vi "Write Custom Serialization Binder Then Read - Returns Same Object.vi"() -> ()   [LabVIEW 2017, in "Generic Object Serializer Tests.lvlib" / "Serialization Binder.lvlib"]
uses:
  Serialization Binder.lvlib
  Generic Object Serializer/Generic Object Serializer.lvclass
  Error Serialization Binder/Error Serialization Binder.lvclass
  C:/Users/de200256/Code/logmanoriginal/jsontext-object-serialization/Serialization Binder/Serialization Binder.lvclass
  Generic Object Serializer/Generic Object Serializer.lvclass/Generic Object Serializer.ctl
  Generic Object Serializer/Write Serialization Binder.vi
  Generic Object Serializer/Read Serialization Binder.vi
  Default Serialization Binder/Default Serialization Binder.lvclass
  Serialization Binder/Serialization Binder.lvclass
  <vilib>/addons/_JKI Toolkits/Caraya/classes/Assert/Assert.lvclass
  <vilib>/addons/_JKI Toolkits/Caraya/classes/Test/Test.lvclass
panel:
  out "error out":errorcluster
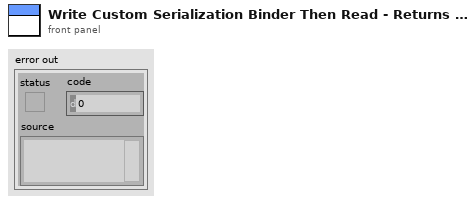
[diagram p1: front panel]
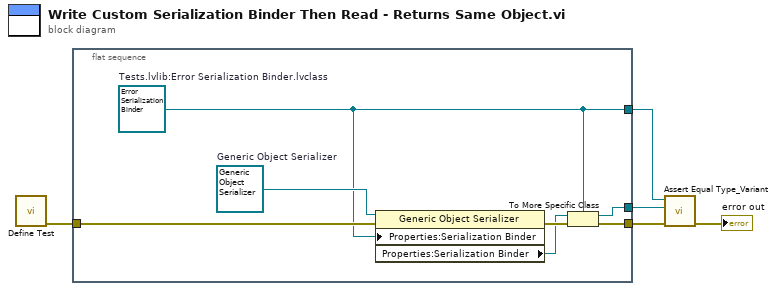
[diagram p0: block diagram]
diagram:
  n1 = call <vilib>:"Define Test.vi"() -> ("error out"=w3:errorcluster)  [unwired: 11 in]
  n2 = flat-sequence {
    tunnel: [w7] -> w5
    tunnel: [w6] -> w4
    tunnel: w3 -> [w11]
    tunnel: [w9] -> w2
    frame #0 {
      w6 = refnum<class "Error Serialization Binder.lvclass"> refnum  # Tests.lvlib:Error Serialization Binder.lvclass
      w12 = refnum<class "Generic Object Serializer.lvclass"> refnum  # Generic Object Serializer
      n3 = property class="Generic Object Serializer"(reference=w12, error in=w11, "Properties:Serialization Binder"=w6) -> (error out=w10:errorcluster, "Properties:Serialization Binder"=w8:refnum<class "Serialization Binder.lvclass">)  [unwired: 1 out]
      n4 = To More Specific Class(target class=w6, reference=w8, error in=w10) -> (specific class reference=w7:refnum<class "Error Serialization Binder.lvclass">, error out=w9:errorcluster)
    }
  }
  n5 = call <vilib>:"Assert Equal Type_Variant.vi"("error in (no error)"=w2, "Y"=w5, "X"=w4) -> ("error out"=→"error out":errorcluster)  [unwired: 8 in]
